vi "OSPEC-Open-Ocean.vi"(8 "Integration Time":i32, 11 "delay":i32) -> (0 "WL Values":dbl[](array[numeric]), 2 "Wrapper Out":u32, 3 "ContinuousStrobe Out":u32)   [LabVIEW 2022 SP3]
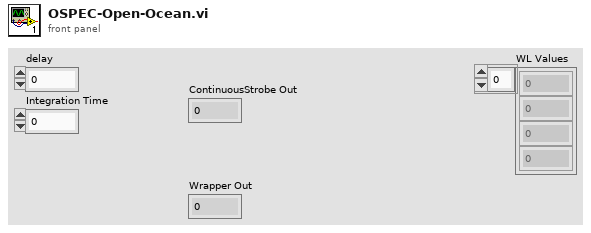
[diagram p1: front panel]
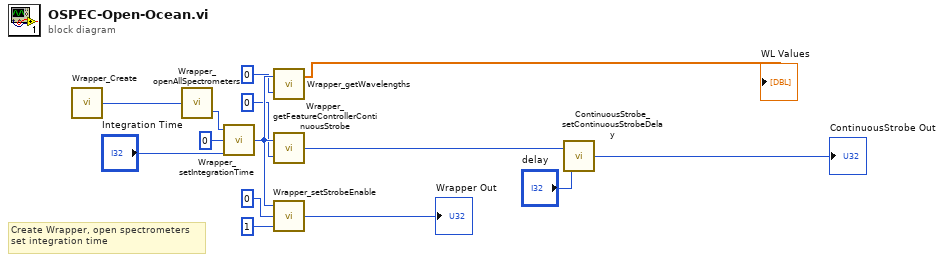
[diagram p0: block diagram]
diagram:
  # "Create Wrapper, open spectrometers\nset integration time"
  n1 = call "Wrapper_Create.vi"() -> ("Wrapper"=w6:u32)
  n2 = call "Wrapper_openAllSpectrometers.vi"("Wrapper In"=w6) -> ("Wrapper Out"=w12:u32)  [unwired: 1 out]
  n3 = call "Wrapper_setIntegrationTime.vi"("Integration Time"="Integration Time", "Spectrometer Index"=0 ("Index"), "Wrapper In"=w12) -> ("Wrapper Out"=w14:u32)
  n4 = call "Wrapper_getWavelengths.vi"("Index"=0, "Wrapper"=w14) -> ("WL Values"=→"WL Values":dbl[])  [unwired: 1 out]
  n5 = call "Wrapper_getFeatureControllerContinuousStrobe.vi"("Index"=0, "Wrapper"=w14) -> ("ContinuousStrobe"=w9:u32)
  n6 = call "Wrapper_setStrobeEnable.vi"("On/Off"=1, "Index"=0, "Wrapper In"=w14) -> ("Wrapper Out"=→"Wrapper Out":u32)
  n7 = call "ContinuousStrobe_setContinuousStrobeDelay.vi"("delay"="delay", "ContinuousStrobe In"=w9) -> ("ContinuousStrobe Out"=→"ContinuousStrobe Out":u32)
